vi "Choose EQ to load.vi"(2 "EQ folders":string[](array[string])) -> (5 "I Leakage":u8, 6 "HV last value":i16, 7 "loaded EQ folder":string)   [LabVIEW 2015, in "VIPM2.lvlib"]
doc: "Obre una finestra emergent amb la llista de Equalitzacions per triar-ne una."
uses:
  VIPM2.lvlib
panel:
  in  "List":cluster{"Button":bool, "EQ execution":string}[](array[cluster])
  # "Choose the Equalization to load"
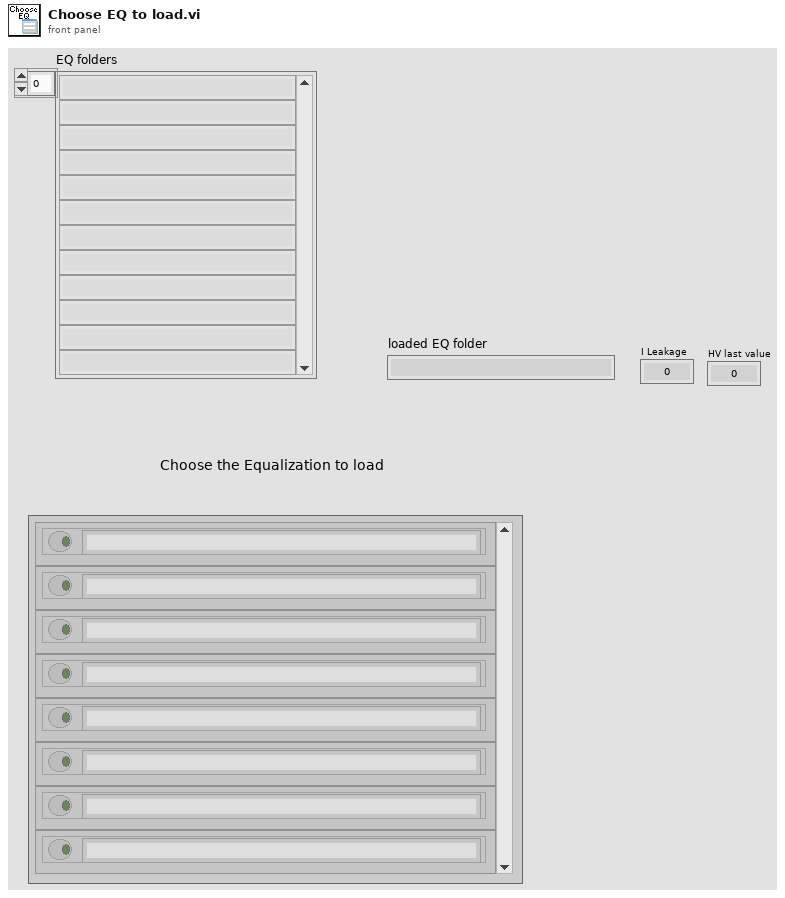
[diagram p1: front panel]
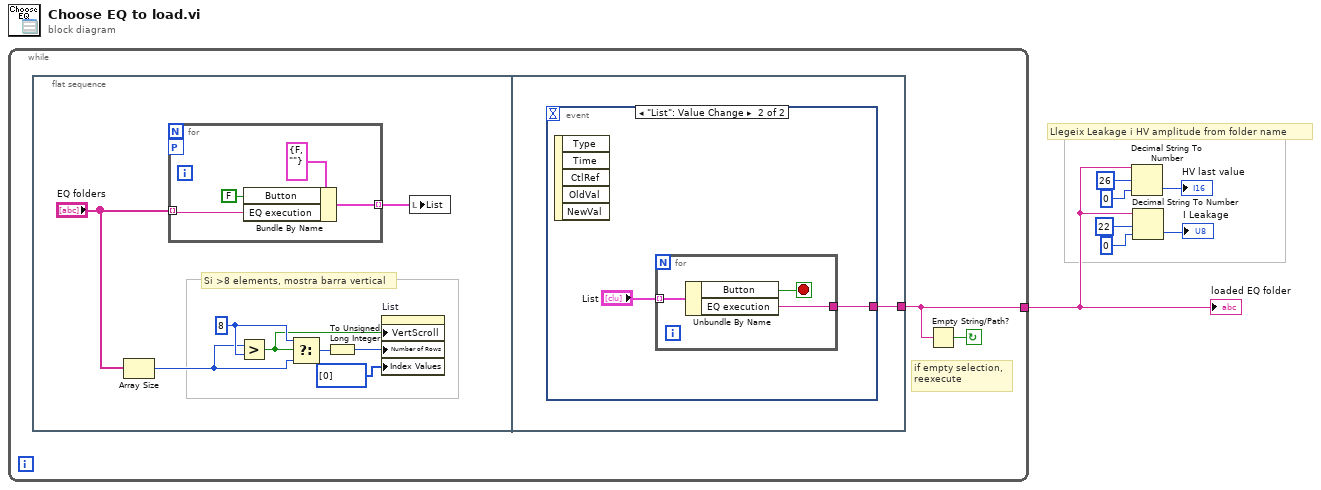
[diagram p0: block diagram]
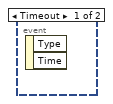
[diagram p2: hidden frame]
diagram:
  # "Llegeix Leakage i HV amplitude from folder name"
  n1 = while {
    tunnel: [w8] -> w1
    stop <- w9 continue-if-true
    # "if empty selection,\nreexecute"
    n2 = flat-sequence {
      tunnel: [w22] -> w8
      frame #0 {
        w17 = 8 ("y")
        # "Si >8 elements, mostra barra vertical"
        n3 = Array Size(array="EQ folders") -> (size(s)=w16:i32)
        n4 = for {
          tunnel: "EQ folders" -> [w20] mode=indexing
          tunnel: [w19] -> w11 mode=indexing
          workers-P: _ -> [_]
          n5 = Bundle By Name(cluster=cluster{"Button":bool, "EQ execution":string} {"Button"=FALSE, "EQ execution"=""} ("Cluster"), "Button"=FALSE, "EQ execution"=w20) -> (w19:cluster{"Button":bool, "EQ execution":string})
        }
        n6 = Greater?(x=w16, y=w17) -> (0:w15:bool)
        n7 = Select(t=w17, s=w15, f=w16) -> (s? t:f=w14:i32)
        n8 = To Unsigned Long Integer(number=w14) -> (unsigned 32bit integer=w13:u32)
        n9 = property on="List" class="Arr (strict)"("VertScroll"=w15, "Number of Rows"=w13, "Index Values"=u32[] [0]) -> ()  [unwired: 2 in, 2 out]
        n10 = local write "List"(w11) -> ()
      }
      frame #1 {
        n11 = event shown="[1] \"List\": Value Change" {
          selector: _ -> [_ _]
          dyn-events: _ -> [_ _]
          timeout: _ -> [_ _]
          tunnel: [_ w23] -> w22
          event Timeout {
            n12 = event-data() -> ()  [unwired: 1 in, 2 out]
          }
          event "List": Value Change {
            n13 = event-data() -> ()  [unwired: 1 in, 5 out]
            n14 = for {
              tunnel: "List" -> [w27] mode=indexing
              tunnel: [w25] -> w23
              stop <- w26 stop-if-true
              n15 = Unbundle By Name(w27) -> ("Button"=w26:bool, "EQ execution"=w25:string)
            }
          }
        }
      }
    }
    n16 = Empty String/Path?(string/path=w8) -> (empty?=w9:bool)
  }
  "loaded EQ folder" <- w1
  n17 = Decimal String To Number(string=w1, offset=26 ("offset (0)"), default (0L)=i16 0 ("default (0 I32)")) -> (number=→"HV last value":i16)  [unwired: 1 out]
  n18 = Decimal String To Number(string=w1, offset=22, default (0L)=u8 0 ("default (0 I32)")) -> (number=→"I Leakage":u8)  [unwired: 1 out]
